vi "OpenI2C.vi"(8 "error in (no error)":errorcluster, 9 "Update Rate (4Hz-100Hz)":u8=100, 11 "I2C Bus":T1=enum."Invalid") -> (0 "error out":errorcluster, 3 "navX out":refnum<class "navX.lvclass">)   [LabVIEW 2015, in "navX Library v3.lvlib" / "navX.lvclass"]
uses:
  navX.lvclass
  <vilib>/Rock Robotics/SystemInterfaces/i2clib/i2c_bus.ctl
  navX - I2C/navX - I2C.lvclass
  navX - I2C/navX - I2C.lvclass/navX - I2C.ctl
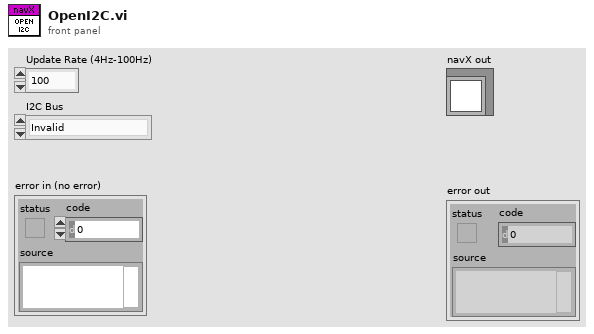
[diagram p1: front panel]
types:
  T1 = typedef "i2c_bus.ctl" = enum16{"I2C On-Board", "I2C MXP", "Invalid"}
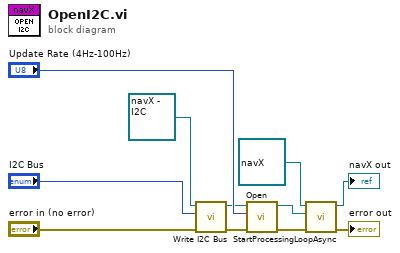
[diagram p0: block diagram]
diagram:
  n1 = call "Write I2C Bus.vi"("error in (no error)"="error in (no error)", "I2C Bus"="I2C Bus", "navX - I2C in"=refnum<class "navX - I2C.lvclass"> refnum ("navX Library v3.lvlib:navX - I2C.lvclass")) -> ("error out"=w8:errorcluster, "navX - I2C out"=w9:refnum<class "navX - I2C.lvclass">)  [unwired: 7 in]
  n2 = call-dynamic "Open.vi"("error in (no error)"=w8, "Update Rate (4Hz-100Hz)"="Update Rate (4Hz-100Hz)", "navX - I2C in"=w9) -> ("error out"=w2:errorcluster, "navX - I2C out"=w5:refnum<class "navX - I2C.lvclass">)  [unwired: 7 in]
  n3 = call "StartProcessingLoopAsync.vi"("error in (no error)"=w2, "navX Class in"=w5, "navX in"=refnum<class "navX.lvclass"> refnum ("navX Library v3.lvlib:navX.lvclass")) -> ("error out"=→"error out":errorcluster, "navX out"=→"navX out":refnum<class "navX.lvclass">)  [unwired: 7 in]
